vi "PH_AWG-510.Trigger Settings Labels.vi"() -> (0 "Trigger Settings Labels":string[](array[string]))   [LabVIEW 2014, in "PH_AWG-510.lvlib"]
uses:
  PH_AWG-510.lvlib
  PH_AWG-510.Trigger Settings.ctl
panel:
  in  "Trigger Settings":T1={"Mode"=enum."Continuous", "Level (V)"=-1.0, "External Source"=FALSE}
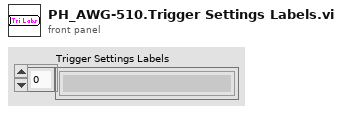
[diagram p1: front panel]
types:
  T1 = typedef "PH_AWG-510.lvlib/PH_AWG-510.Trigger Settings.ctl" = cluster{"Mode":enum16{"Continuous", "Triggered", "Gated", "Enhanced"}, "Level (V)":dbl, "External Source":bool}
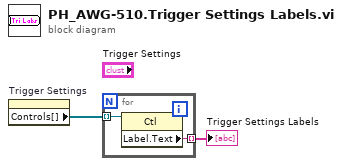
[diagram p0: block diagram]
diagram:
  n1 = property on="Trigger Settings" class="Clust (strict)"() -> ("Controls[]"=w1:refnum<vi>[])  [unwired: 2 in, 2 out]
  n2 = for {
    tunnel: w1 -> [w4] mode=indexing
    tunnel: [w3] -> w2 mode=indexing
    n3 = property class="Ctl"(reference=w4) -> ("Label.Text"=w3:string)  [unwired: 1 in, 2 out]
  }
  "Trigger Settings Labels" <- w2
